vi "TEST - Search or Split String.vi"(8 "error in":errorcluster) -> (0 "error out":errorcluster, 2 "pass":bool)   [LabVIEW 2009]
panel:
  out "Failures":T1(array[cluster])
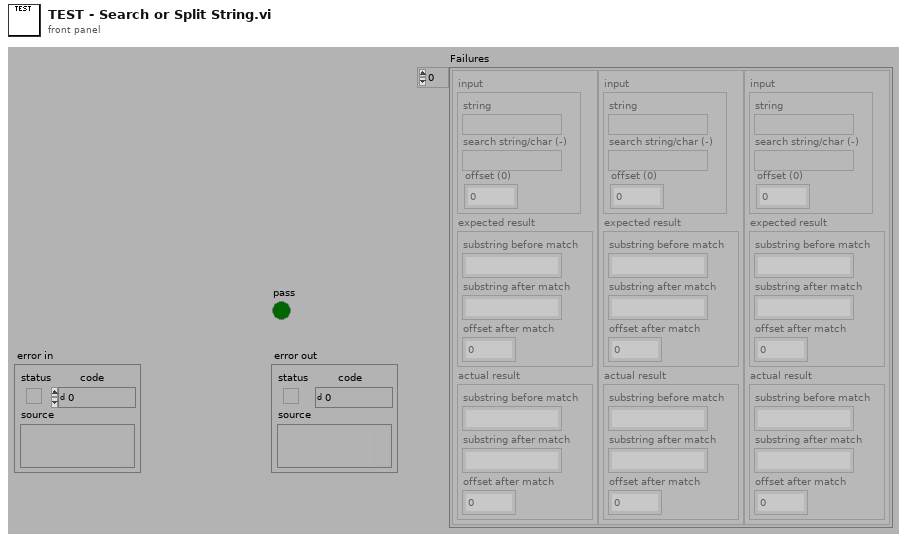
[diagram p1: front panel]
types:
  T1 = cluster{"input":cluster{"string":string, "search string/char (-)":string, "offset (0)":i32}, "expected result":cluster{"substring before match":string, "substring after match":string, "offset after match":i32}, "actual result":cluster{"substring before match":string, "substring after match":string, "offset after match":i32}}[]
  T2 = cluster{"string":string, "search string/char (-)":string, "offset (0)":i32}
  T3 = cluster{"substring before match":string, "substring after match":string, "offset after match":i32}
  T4 = cluster{"input":cluster{"string":string, "search string/char (-)":string, "offset (0)":i32}, "expected result":cluster{"substring before match":string, "substring after match":string, "offset after match":i32}, "actual result":cluster{"substring before match":string, "substring after match":string, "offset after match":i32}}
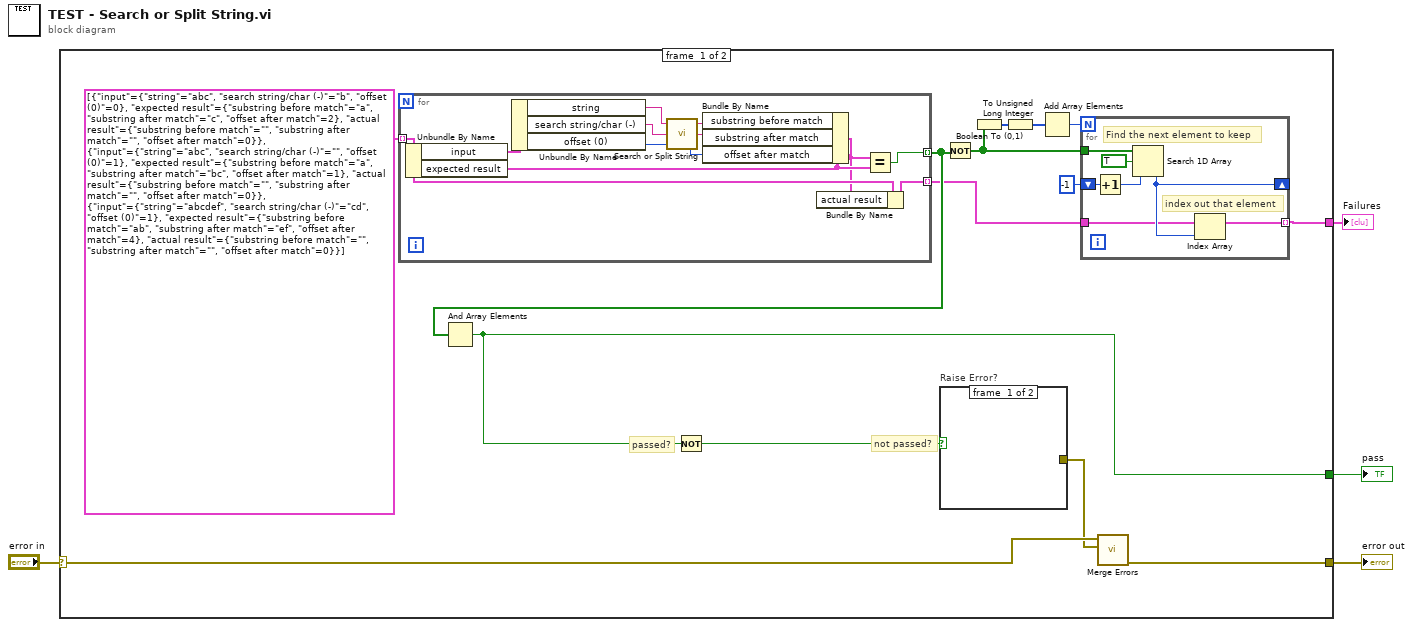
[diagram p0: block diagram]
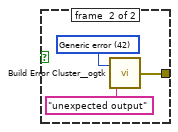
[diagram p2: hidden frame]
diagram:
  n1 = case shown="No Error" "error in" {
    selector: "error in" -> [w18 w41]
    tunnel: [w14 _] -> w4
    tunnel: [w17 w41] -> w2
    tunnel: [w6 _] -> w1
    frame #0 {
      # "not passed?"
      # "passed?"
      n2 = for {
        tunnel: T1 [{"input"={"string"="abc", "search string/char (-)"="b", "offset (0)"=0}, "expected result"={"substring before match"="a", "substring after match"="c", "offset after match"=2}, "actual result"={"substring before match"="", "substring after match"="", "offset after match"=0}}, {"input"={"string"="abc", "search string/char (-)"="", "offset (0)"=1}, "expected result"={"substring before match"="a", "substring after match"="bc", "offset after match"=1}, "actual result"={"substring before match"="", "substring after match"="", "offset after match"=0}}, {"input"={"string"="abcdef", "search string/char (-)"="cd", "offset (0)"=1}, "expected result"={"substring before match"="ab", "substring after match"="ef", "offset after match"=4}, "actual result"={"substring before match"="", "substring after match"="", "offset after match"=0}}] ("Failures") -> [w35] mode=indexing
        tunnel: [w37] -> w8 mode=indexing
        tunnel: [w36] -> w7 mode=indexing
        n3 = Unbundle By Name(w35) -> ("input"=w34:T2, "expected result"=w30:T3)
        n4 = Unbundle By Name(w34) -> ("string"=w33:string, "search string/char (-)"=w32:string, "offset (0)"=w31:i32)
        n5 = call "Search or Split String.vi"("offset (0)"=w31, "search string/char (-)"=w32, "string"=w33) -> ("offset after match"=w27:i32, "substring after match"=w28:string, "substring before match"=w29:string)
        n6 = Bundle By Name(cluster=w30, "substring before match"=w29, "substring after match"=w28, "offset after match"=w27) -> (w26:T3)
        n7 = Bundle By Name(cluster=w35, "actual result"=w26) -> (w36:T4)
        n8 = Equal?(x=w26, y=w30) -> (x = y?=w37:bool)
      }
      n9 = And Array Elements(Boolean array=w8) -> (logical AND=w14:bool)
      n10 = Not(x=w14) -> (.not. x?=w15:bool)
      n11 = case "Raise Error?" shown="True" w15 {
        tunnel: [_ w38] -> w16
        frame #0 {
        }
        frame #1 {
          w39 = 42 items=["No error", "Argument error", "Memory is full", "Out of zone", "End of file", "File already open", "Generic file I/O error", "File not found", "File permission error", "Disk is full", "Duplicate path", "Too many files open", "System feature not enabled", "Resource file not found", "Cannot add resource", "Resource not found", "Image not found", "Image memory error", "Pen does not exist", "Config type invalid", "Config token not found", "Config parse error", "Config memory error", "Bad external code format", "Bad external code offset", "External code not present", "Null window", "Destroy window error", "Null menu", "Print aborted", "Bad print record", "Print driver error", "Windows error during printing", "Memory error during printing", "Print dialog error", "Generic print error", "Invalid device refnum", "Device not found", "Device parameter error", "Device unit error", "Cannot open device", "Device call aborted", "Generic error", "Cancelled by user", "Object ID too low", "Object ID too high", "Object not in heap", "Unknown heap", "Unknown object (invalid DefProc)", "Unknown object (DefProc not in table)", "Message out of range", "Invalid (null) method", "Unknown message", "Manager call not supported", "Bad address", "Network operation in progress", "Network operation timed out", "Connection is busy", "Network attribute not supported", "Network error", "Address in use", "System out of memory", "Connection aborted", "Connection refused", "Not connected", "Already connected", "Connection closed", "Initialization error (interapplication manager)", "Bad occurrence", "Wait on unbound occurrence handler", "Occurrence queue overflow", "Datalog type conflict", "Unused", "Unrecognized type (interapplication manager)", "Memory corrupt", "Failed to make temporary DLL", "Old CIN version", "Drag socket not found", "Failed to load drop-object", "Failed to register OLE object", "Failed to release OLE object", "Format specifier type mismatch", "Unknown format specifier", "Too few format specifiers", "Too many format specifiers", "Scan failed", "Newer CIN version", "Error converting to variant", "Runtime menu error", "Password tampered", "Variant attribute not found", "Incompatible variant data type", "Event data is not available", "Event Store is not present", "Occurrence is not found", "Event Queue is not created", "Event info is not available", "Refnum passed is NULL", "Error retrieving Class GUID", "Error retrieving CoClass GUID", "Error retrieving TypeLib GUID.", "Bad built application magic bytes.", "Specific driver is different from the specific driver associated with the Logical Name.", "There is no session opened to the class driver.", "Max Error", "MAX - Error with config objects", "MAX - Error loading configuration", "MAX - Group not supported"]
          n12 = call <userlib>:"Build Error Cluster__ogtk.vi"("String to Prepend to source (\"\")"="unexpected output" ("String to Prepend to source (\"\")"), "code"=w39) -> ("error out"=w38:errorcluster)
        }
      }
      n13 = Not(x=w8) -> (.not. x?=w10:bool[])
      n14 = Boolean To (0,1)(Boolean=w10) -> (0, 1=w11:i16[])
      n15 = To Unsigned Long Integer(number=w11) -> (unsigned 32bit integer=w9:u32[])
      n16 = Add Array Elements(numeric array=w9) -> (sum=w12:u32)
      n17 = for {
        N: w12 -> [_]
        tunnel: w7 -> [w21]
        tunnel: w10 -> [w25]
        shift-right: [w22] -> _
        shift-left: -1 ("start index (0)") -> [w23]
        tunnel: [w20] -> w6 mode=indexing
        # "index out that element"
        # "Find the next element to keep"
        n18 = Increment(x=w23) -> (x+1=w19:i32)
        n19 = Search 1D Array(1D array=w25, element=TRUE, start index (0)=w19) -> (index of element=w22:i32)
        n20 = Index Array(array=w21, index=w22) -> (element=w20:T4)
      }
      n21 = call <vilib>:"Merge Errors.vi"("error in 2 (no error)"=w16, "error in 1 (no error)"=w18) -> ("error out"=w17:errorcluster)  [unwired: 5 in]
    }
    frame #1 {
    }
  }
  "pass" <- w4
  "error out" <- w2
  "Failures" <- w1
